vi "sub_Gslam_motion-model.vi"(10 "u":T1, 11 "x_true":T1) -> (3 "x_true out":T1)   [LabVIEW 2019]
uses:
  <vilib>/Analysis/Matrix/Datatypes/RealMatrix.ctl
  Ctrl/cmd_common.ctl
  <vilib>/Analysis/Matrix/Numeric/Multiply/Multiply - RM,RM.vi
  <vilib>/Analysis/Matrix/Numeric/Add/Add - RM,RM.vi
  <vilib>/Analysis/Matrix/NI_Matrix.lvlib
panel:
  out "열 x_true":i32
  out "행 x_true":i32
  out "B":T1
  out "행 F":i32
  out "열 F":i32
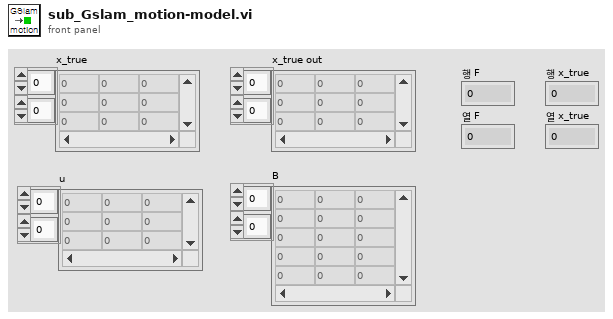
[diagram p1: front panel]
types:
  T1 = typedef "NI_Matrix.lvlib/RealMatrix.ctl" = dbl[][]
  T2 = typedef "cmd_common.ctl" = enum16{"read", "write"}
  T3 = cluster{"Q Sim":T1, "R Sim":T1, "DT":dbl, "SIM_TIME":dbl, "MAX_RANGE":dbl, "STATE_SIZE":i32, "C_SIGMA 1":dbl, "C_SIGMA 2":dbl, "C_SIGMA 3":dbl, "MAX_ITR":u32}
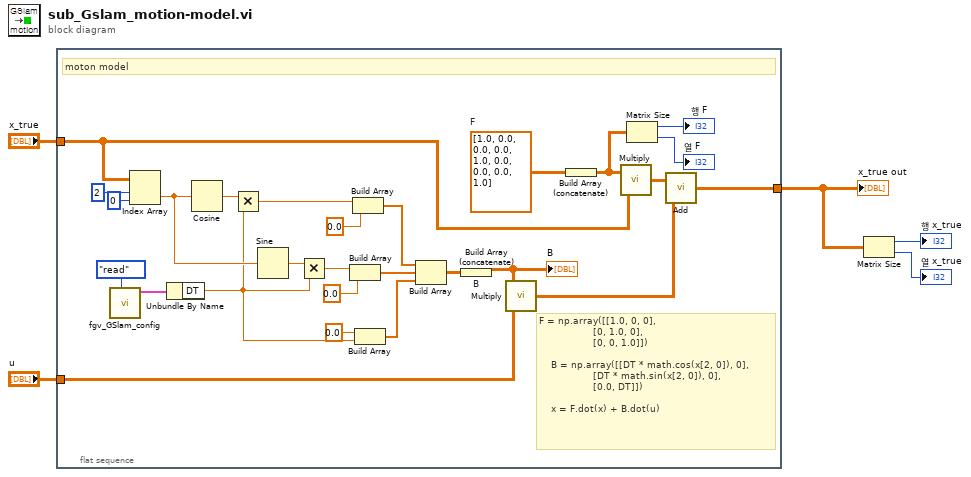
[diagram p0: block diagram]
diagram:
  n1 = flat-sequence {
    tunnel: "x_true" -> [w15]
    tunnel: "u" -> [w13]
    tunnel: [w11] -> w1
    frame #0 {
      w16 = dbl[][] [[1.0, 0.0, 0.0], [0.0, 1.0, 0.0], [0.0, 0.0, 1.0]]  # F
      # "F = np.array([[1.0, 0, 0],\n                  [0, 1.0, 0],\n                  [0, 0, 1.0]])\n\n    B = np.array([[DT * math.cos(x[2, 0]), 0],\n                  [DT * math.sin(x[2, 0]), 0],\n                  [0.0, DT]])\n\n    x = F.dot(x) + B.dot(u)"
      # "moton model"
      n2 = call "fgv_GSlam_config.vi"("cmd"=cmd_common."read") -> ("G cofnig out"=w6:T3)  [unwired: 10 in]
      n3 = Index Array(array=w15, index (row)=2 ("인덱스 (행)"), index (col)=0 ("인덱스 (열)")) -> (element=w28:dbl)
      n4 = Unbundle By Name(w6) -> ("DT"=w12:dbl)
      n5 = Cosine(x=w28) -> (cos(x)=w30:dbl)
      n6 = Multiply(x=w30, y=w12) -> (x*y=w27:dbl)
      n7 = Sine(x=w28) -> (sin(x)=w29:dbl)
      n8 = Multiply(x=w29, y=w12) -> (x*y=w24:dbl)
      n9 = Build Array(w24, 0.0 ("원소")) -> (w21:dbl[])
      n10 = Build Array(w27, 0.0 ("원소")) -> (w20:dbl[])
      n11 = Build Array(0.0 ("원소"), w12) -> (w22:dbl[])
      n12 = Build Array(w20, w21, w22) -> (w19:dbl[][])
      n13 = Build Array (concatenate) "B"(w19) -> (w18:T1)
      "B" <- w18
      n14 = call-poly <vilib>:"Multiply.vi"("Real Matrix B"=w13, "Real Matrix A"=w18) -> ("A * B"=w17:T1)
      n15 = Build Array (concatenate)(w16) -> (w10:T1)
      n16 = call-poly <vilib>:"Multiply.vi"("Real Matrix B"=w15, "Real Matrix A"=w10) -> ("A * B"=w14:T1)
      n17 = Matrix Size(0:w10) -> (1:→"행 F":i32, 2:→"열 F":i32)
      n18 = call-poly <vilib>:"Add.vi"("Real Matrix B"=w17, "Real Matrix A"=w14) -> ("A + B"=w11:T1)
    }
  }
  n19 = Matrix Size(0:w1) -> (1:→"행 x_true":i32, 2:→"열 x_true":i32)
  "x_true out" <- w1
